vi "setunitfornumber.vi"(10 "Einheit":string, 11 "Numeric":dbl) -> (3 "String":string)   [LabVIEW 2013, in "EMV-Test.lvlib"]
uses:
  EMV-Test.lvlib
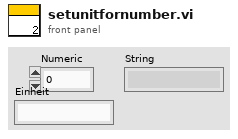
[diagram p1: front panel]
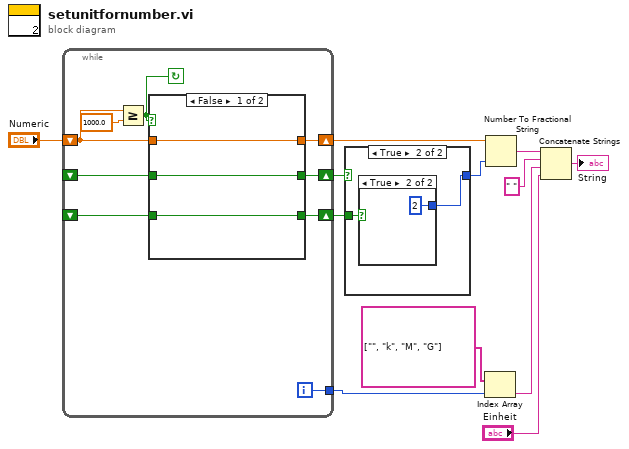
[diagram p0: block diagram]
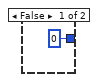
[diagram p2: hidden frame]
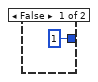
[diagram p3: hidden frame]
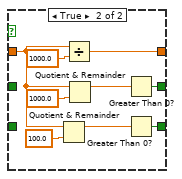
[diagram p4: hidden frame]
diagram:
  n1 = while {
    shift-right: [w20] -> w11
    shift-left: "Numeric" -> [w18]
    tunnel: [w21] -> w9
    shift-right: [w17] -> w3
    shift-left: _ -> [w15]
    shift-right: [w16] -> w2
    shift-left: _ -> [w14]
    i -> [w21]
    stop <- w19 continue-if-true
    n2 = Greater Or Equal?(x=w18, y=1000.0) -> (x >= y?=w19:bool)
    n3 = case shown="False" w19 {
      tunnel: w18 -> [w22 w25]
      tunnel: [w22 w26] -> w20
      tunnel: [w24 w29] -> w17
      tunnel: [w23 w28] -> w16
      tunnel: w15 -> [w24 _]
      tunnel: w14 -> [w23 _]
      frame False {
      }
      frame True {
        n4 = Quotient & Remainder(x=w25, y=100.0) -> (x-y*floor(x/y)=w33:dbl)  [unwired: 1 out]
        n5 = Divide(x=w25, y=1000.0) -> (x/y=w26:dbl)
        n6 = Quotient & Remainder(x=w25, y=1000.0) -> (x-y*floor(x/y)=w31:dbl)  [unwired: 1 out]
        n7 = Greater Than 0?(x=w31) -> (x > 0?=w29:bool)
        n8 = Greater Than 0?(x=w33) -> (x > 0?=w28:bool)
      }
    }
  }
  n9 = case shown="True" w3 {
    tunnel: w2 -> [_ w36]
    tunnel: [i16 0 ("precision (6)") w35] -> w1
    frame False {
    }
    frame True {
      n10 = case shown="True" w36 {
        tunnel: [i16 1 ("precision (6)") i16 2 ("precision (6)")] -> w35
        frame False {
        }
        frame True {
        }
      }
    }
  }
  n11 = Index Array(array=string[] ["", "k", "M", "G"], index=w9) -> (element=w6:string)
  n12 = Number To Fractional String(number=w11, precision (6)=w1) -> (F-format string=w10:string)  [unwired: 2 in]
  n13 = Concatenate Strings(w10, " " ("string"), w6, "Einheit") -> (→"String":string)
